vi "GetHWI.vi"(8 "error in (no error)":errorcluster, 11 "Novatech in":refnum<class "Novatech.lvclass">) -> (0 "error out":errorcluster, 2 "Novatech Hardware Image":T1, 3 "Novatech out":refnum<class "Novatech.lvclass">)   [LabVIEW 2013, in "Novatech.lvclass"]
uses:
  Novatech.lvclass
  Novatech.lvclass/Novatech.ctl
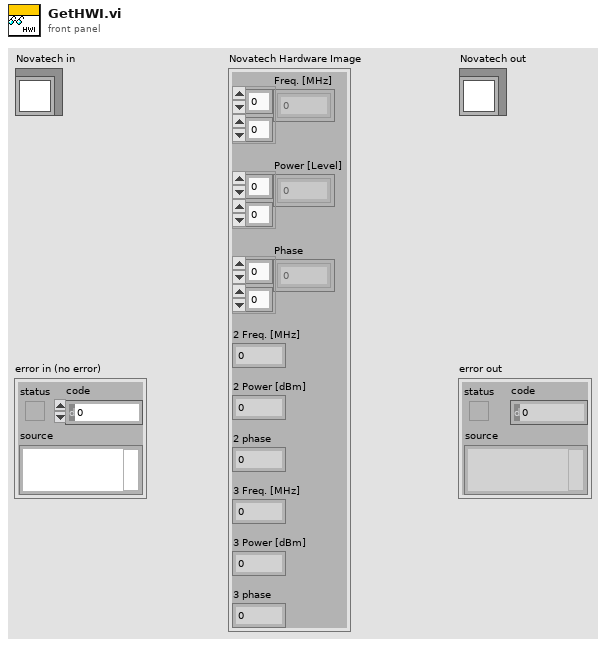
[diagram p1: front panel]
types:
  T1 = cluster{"Freq. [MHz]":dbl[][], "Power [Level]":u16[][], "Phase":u16[][], "2 Freq. [MHz]":dbl, "2 Power [dBm]":u16, "2 phase":u16, "3 Freq. [MHz]":dbl, "3 Power [dBm]":u16, "3 phase":u16}
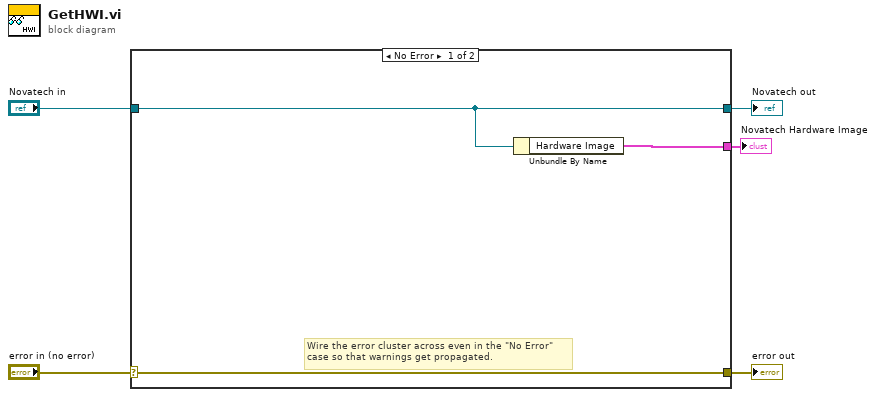
[diagram p0: block diagram]
diagram:
  n1 = case shown="No Error" "error in (no error)" {
    selector: "error in (no error)" -> [w8 w10]
    tunnel: [w8 w10] -> w4
    tunnel: [w7 w9] -> w2
    tunnel: "Novatech in" -> [w7 w9]
    tunnel: [w6 _] -> w1
    frame No Error {
      # "Wire the error cluster across even in the \"No Error\"\ncase so that warnings get propagated."
      n2 = Unbundle By Name(w7) -> ("Hardware Image"=w6:T1)
    }
    frame Error {
    }
  }
  "error out" <- w4
  "Novatech out" <- w2
  "Novatech Hardware Image" <- w1
